vi "Test scriere I2C.vi"(8 "error in (no error)":errorcluster, 9 "use7bitAddress":bool, 10 "i2cTxData":u8[](array[numeric])=[0, 7], 11 "slaveAddress":u8=188 format="%.0b") -> (0 "error out":errorcluster, 2 "handle out":u64, 3 "noOfDevs out":u32=1)   [LabVIEW 2020]
uses:
  mcp2221_dll_um_x64.dll
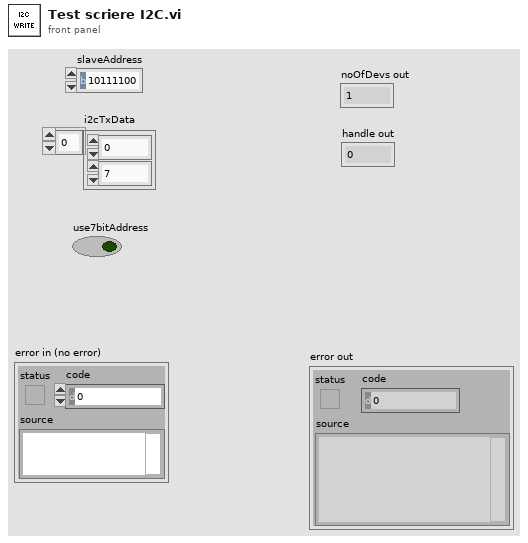
[diagram p1: front panel]
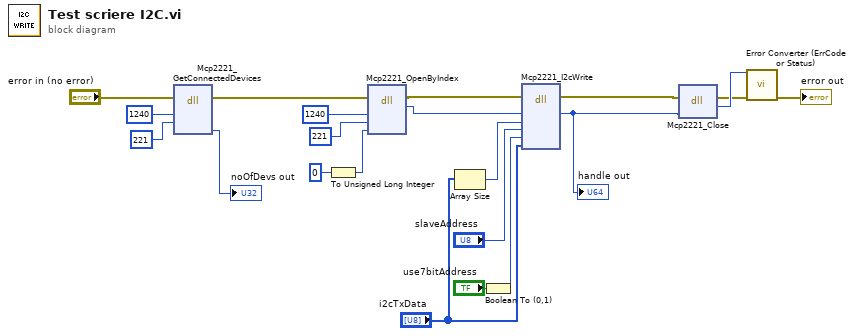
[diagram p0: block diagram]
diagram:
  n1 = dll-call lib="C:/Users/tuguialexand/Desktop/Licenta/MCP2221A LabVIEW library/Microchip MCP2221A_64bit/VIs/Private/mcp2221_dll_um_x64.dll" fn="Mcp2221_GetConnectedDevices"(error in="error in (no error)", "vid"=u32 1240, "pid"=u32 221) -> (error out=w12:errorcluster, "noOfDevs"=→"noOfDevs out":u32)  [unwired: 6 in, 1 out]
  n2 = To Unsigned Long Integer(number=0 ("index")) -> (unsigned 32bit integer=w15:u32)
  n3 = dll-call lib="C:/Users/tuguialexand/Desktop/Licenta/MCP2221A LabVIEW library/Microchip MCP2221A_64bit/VIs/Private/mcp2221_dll_um_x64.dll" fn="Mcp2221_OpenByIndex"(error in=w12, "VID"=u32 1240, "PID"=u32 221, "index"=w15) -> (error out=w4:errorcluster, "return type"=w1:u64)  [unwired: 5 in, 1 out]
  n4 = Array Size(array="i2cTxData") -> (size(s)=w5:i32)
  n5 = Boolean To (0,1)(Boolean="use7bitAddress") -> (0, 1=w7:i16)
  n6 = dll-call lib="C:/Users/tuguialexand/Desktop/Licenta/MCP2221A LabVIEW library/Microchip MCP2221A_64bit/VIs/Private/mcp2221_dll_um_x64.dll" fn="Mcp2221_I2cWrite"(error in=w4, "handle"=w1, "bytesToWrite"=w5, "slaveAddress"="slaveAddress", "use7bitAddress"=w7, "i2cTxData"="i2cTxData") -> (error out=w3:errorcluster, "handle"=w2:u64)  [unwired: 7 in, 1 out]
  "handle out" <- w2
  n7 = dll-call lib="C:/Users/tuguialexand/Desktop/Licenta/MCP2221A LabVIEW library/Microchip MCP2221A_64bit/VIs/Private/mcp2221_dll_um_x64.dll" fn="Mcp2221_Close"(error in=w3, "handle"=w2) -> (error out=w10:errorcluster, "return type"=w11:i32)  [unwired: 3 in, 1 out]
  n8 = call "Error Converter (ErrCode or Status).vi"("error code"=w11, "error in (no error)"=w10) -> ("error out"=→"error out":errorcluster)  [unwired: 13 in]
